vi "Handle Analog Commands.vi"(8 "error in (no error)":errorcluster, 10 "Commands":T1, 11 "DAQmxAO in":refnum<class "DAQmxAO.lvclass">) -> (0 "error out":errorcluster, 3 "DAQmxAO out":refnum<class "DAQmxAO.lvclass">)   [LabVIEW 2023, in "VolatusDAQ.lvlib" / "DAQmxAO.lvclass"]
uses:
  DAQmxAO.lvclass
  DAQmxAO.lvclass/DAQmxAO.ctl
  lv-vecto/Vecto/Group DBL/Group DBL.lvclass
  lv-vecto/Vecto/Group/Group.lvclass
  VolatusData/Scaling/Scaling.lvclass
  Volatus/Module/Module.lvclass
  <vilib>/DAQmx/write.llb/DAQmx Write (Analog 1D DBL NChan 1Samp).vi
  C:/dev/volatus/mts-volatus-super/libs/lv-vecto/Vecto/Group/Group.lvclass
  C:/dev/volatus/mts-volatus-super/libs/lv-vecto/Vecto/Group DBL/Group DBL.lvclass
  C:/dev/volatus/mts-volatus-super/libs/lv-volatus/Volatus/Module/Module.lvclass
  C:/dev/volatus/mts-volatus-super/libs/lv-volatus/VolatusDAQ/DAQmxAO/DAQmxAO.lvclass
  messages/CmdAnalog/Data.ctl
  messages/CmdAnalog/CmdAnalog.lvlib
  messages/CmdAnalogMultiple/Data.ctl
  messages/CmdAnalogMultiple/CmdAnalogMultiple.lvlib
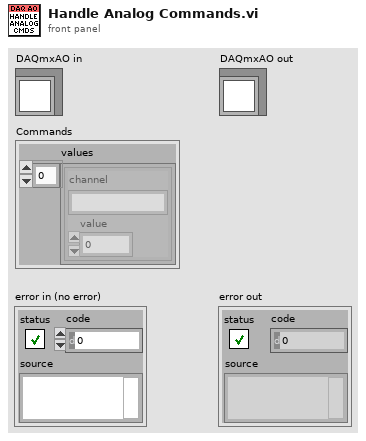
[diagram p1: front panel]
types:
  T1 = typedef "CmdAnalogMultiple.lvlib/Data.ctl" = cluster{"values":T2[]}
  T2 = typedef "CmdAnalog.lvlib/Data.ctl" = cluster{"channel":string, "value":dbl}
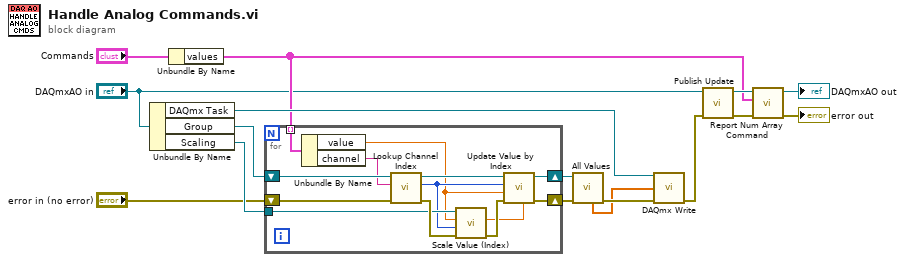
[diagram p0: block diagram]
diagram:
  n1 = Unbundle By Name("DAQmxAO in") -> ("DAQmx Task"=w10:refnum<k21>, "Group"=w16:refnum<class "Group DBL.lvclass">, "Scaling"=w15:refnum<class "Scaling.lvclass">)
  n2 = Unbundle By Name("Commands") -> ("values"=w6:T2[])
  n3 = for {
    tunnel: w15 -> [w25]
    shift-right: [w21] -> w14
    shift-left: "error in (no error)" -> [w28]
    shift-right: [w20] -> w13
    shift-left: w16 -> [w27]
    tunnel: w6 -> [w19] mode=indexing
    n4 = Unbundle By Name(w19) -> ("value"=w17:dbl, "channel"=w18:string)
    n5 = call "Lookup Channel Index.vi"("error in (no error)"=w28, "Channel Name"=w18, "Group in"=w27) -> ("error out"=w29:errorcluster, "Index"=w24:i32, "Group out"=w26:refnum<class "Group DBL.lvclass">)  [unwired: 6 in]
    n6 = call "Scale Value (Index).vi"("error in (no error)"=w29, "Index"=w24, "Value"=w17, "VolatusScaling in"=w25) -> ("error out"=w23:errorcluster, "Scaled Value"=w22:dbl)  [unwired: 5 in, 1 out]
    n7 = call "Update Value by Index.vi"("Raw"=w22, "error in (no error)"=w23, "Scaled"=w17, "Index"=w24, "Group in"=w26) -> ("error out"=w21:errorcluster, "Group out"=w20:refnum<class "Group DBL.lvclass">)  [unwired: 5 in]
  }
  n8 = call "All Values.vi"("error in (no error)"=w14, "Group in"=w13) -> ("error out"=w12:errorcluster, "Raw"=w11:dbl[])  [unwired: 5 in, 3 out]
  n9 = call-poly <vilib>:"DAQmx Write.vi"("task/channels in"=w10, "data"=w11, "error in"=w12) -> ("error out"=w9:errorcluster)  [unwired: 10 in, 2 out]
  n10 = call "Publish Update.vi"("error in (no error)"=w9, "DAQmxAO in"="DAQmxAO in") -> ("error out"=w8:errorcluster, "DAQmxAO out"=w7:refnum<class "DAQmxAO.lvclass">)  [unwired: 8 in]
  n11 = call "Report Num Array Command.vi"("error in (no error)"=w8, "Command"=w6, "Module in"=w7) -> ("error out"=→"error out":errorcluster, "Module out"=→"DAQmxAO out":refnum<class "DAQmxAO.lvclass">)  [unwired: 7 in]
